vi "TestIntegration.vi"() -> ()   [LabVIEW 2019]
uses:
  ParseVectorFile/Typedefs/PublicEvents--ParseVectorFile.ParsedData.ctl
  Image/SVGImage.lvclass
  ParsePaths/Path.lvclass
  Rectangle/Rectangle.lvclass
  Dot/Dot.lvclass
  PathCommands/Point.ctl
  ParseVectorFile/ParseVectorFile.lvclass
  C:/Program Files (x86)/National Instruments/LabVIEW 2019/vi.lib/JKI/JKI SMO/SMO/SMO.lvclass
  ParsePaths/Path.lvclass/Path.ctl
  ParsePaths/Read Path Commands.vi
  PathCommands/PathCommands.lvclass
  <vilib>/JKI/JKI SMO/SMO/SMO.lvclass
panel:
  out "Points":T1[](array[typedef])
  out "xml string":string
  out "ParsedData":T2
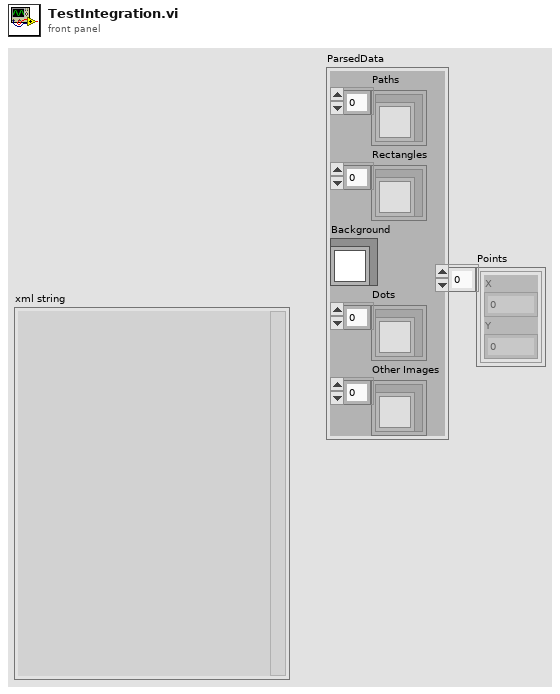
[diagram p1: front panel]
types:
  T1 = typedef "PathCommands.lvclass/Point.ctl" = cluster{"X":dbl, "Y":dbl}
  T2 = typedef "ParseVectorFile.lvclass/PublicEvents--ParseVectorFile.ParsedData.ctl" = cluster{"Paths":refnum<class "Path.lvclass">[], "Rectangles":refnum<class "Rectangle.lvclass">[], "Background":refnum<class "SVGImage.lvclass">, "Dots":refnum<class "Dot.lvclass">[], "Other Images":refnum<class "SVGImage.lvclass">[]}
  T3 = enum16{"open", "replace", "create", "open or create", "replace or create", "replace or create with confirmation"}
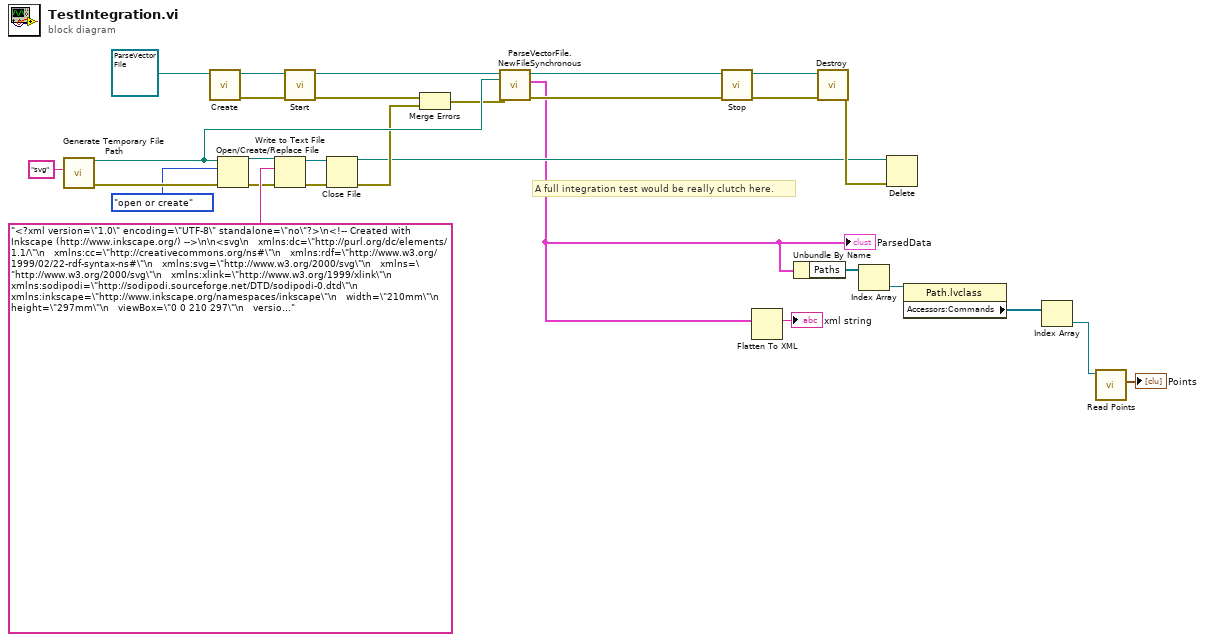
[diagram p0: block diagram]
diagram:
  # "A full integration test would be really clutch here."
  n1 = call <vilib>:"Generate Temporary File Path.vi"("Temporary File Extension (tmp)"="svg") -> ("error out"=w26:errorcluster, "Unique Temporary File Path"=w18:path)  [unwired: 9 in]
  n2 = call <vilib>:"Create.vi"("SMO"=refnum<class "ParseVectorFile.lvclass"> refnum ("ParseVectorFile.lvclass")) -> ("error out"=w14:errorcluster, "SMO out"=w21:refnum<class "ParseVectorFile.lvclass">)  [unwired: 8 in, 1 out]
  n3 = Open/Create/Replace File(file path (use dialog)=w18, error in=w26, operation (0:open)=T3."open or create") -> (refnum out=w24:refnum<file>, error out=w25:errorcluster)  [unwired: 3 in, 1 out]
  n4 = Write to Text File(file (use dialog)=w24, text="<?xml version=\"1.0\" encoding=\"UTF-8\" standalone=\"no\"?>\n<!-- Created with Inkscape (http://www.inkscape.org/) -->\n\n<svg\n   xmlns:dc=\"http://purl.org/dc/elements/1.1/\"\n   xmlns:cc=\"http://creativecommons.org/ns#\"\n   xmlns:rdf=\"http://www.w3.org/1999/02/22-rdf-syntax-ns#\"\n   xmlns:svg=\"http://www.w3.org/2000/svg\"\n   xmlns=\"http://www.w3.org/2000/svg\"\n   xmlns:xlink=\"http://www.w3.org/1999/xlink\"\n   xmlns:sodipodi=\"http://sodipodi.sourceforge.net/DTD/sodipodi-0.dtd\"\n   xmlns:inkscape=\"http://www.inkscape.org/namespaces/inkscape\"\n   width=\"210mm\"\n   height=\"297mm\"\n   viewBox=\"0 0 210 297\"\n   version=\"1.1\"\n   id=\"svg8\"\n   inkscape:version=\"0.92.4 (5da689c313, 2019-01-14)\"\n   sodipodi:docname=\"Rotated Rectangle.svg\">\n  <defs\n     id=\"defs2\" />\n  <sodipodi:namedview\n     id=\"base\"\n     pagecolor=\"#ffffff\"\n     bordercolor=\"#666666\"\n     borderopacity=\"1.0\"\n     inkscape:pageopacity=\"0.0\"\n     inkscape:pageshadow=\"2\"\n     inkscape:zoom=\"1.979899\"\n     inkscape:cx=\"401.06977\"\n     inkscape:cy=\"632.73714\"\n     inkscape:document-units=\"mm\"\n     inkscape:current-layer=\"layer1\"\n     showgrid=\"false\"\n     inkscape:window-width=\"1920\"\n     inkscape:window-height=\"1001\"\n     inkscape:window-x=\"-9\"\n     inkscape:window-y=\"-9\"\n     inkscape:window-maximized=\"1\" />\n  <metadata\n     id=\"metadata5\">\n    <rdf:RDF>\n      <cc:Work\n         rdf:about=\"\">\n        <dc:format>image/svg+xml</dc:format>\n        <dc:type\n           rdf:resource=\"http://purl.org/dc/dcmitype/StillImage\" />\n        <dc:title />\n      </cc:Work>\n    </rdf:RDF>\n  </metadata>\n  <g\n     inkscape:label=\"Layer 1\"\n     inkscape:groupmode=\"layer\"\n     id=\"layer1\">\n    <rect\n       style=\"opacity:1;fill:#00ff00;fill-opacity:1;stroke:#000000;stroke-width:0.2;stroke-miterlimit:4;stroke-dasharray:none;stroke-opacity:1\"\n       id=\"rect10\"\n       width=\"10.1\"\n       height=\"10.2\"\n       x=\"-10.3\"\n       y=\"10.4\"\n       transform=\"rotate(-10.5)\" />\n    <rect\n       style=\"opacity:1;fill:#00ff00;fill-opacity:1;stroke:#000000;stroke-width:0.2;stroke-miterlimit:4;stroke-dasharray:none;stroke-opacity:1\"\n       id=\"rect12\"\n       width=\"10.6\"\n       height=\"10.7\"\n       x=\"-10.8\"\n       y=\"10.9\"\n       inkscape:transform-center-x=\"33.251622\"\n       inkscape:transform-center-y=\"66.085109\"\n       transform=\"rotate(-11.1)\" />\n    <image\n       sodipodi:absref=\"C:\\gold_75nm_low_voltage.png\"\n       y=\"100.1\"\n       x=\"100\"\n       id=\"image33\"\n       xlink:href=\"file:///C:/gold_75nm_low_voltage.png\"\n       preserveAspectRatio=\"none\"\n       height=\"70.1\"\n       width=\"70\" />\n    <path\n       style=\"fill:none;stroke:#45fc03;stroke-width:0.123456789px;stroke-linecap:butt;stroke-linejoin:miter;stroke-opacity:1\"\n       d=\"m 1.1,1.2 c 1.3,1.4 1.5,-1.6 1.7,-1.8 1.9,1.10 1.11,1.12 1.13,1.14 0,0 1.15,1.16 1.17,1.18 -1.19,1.20 -1.21,-1.22 -1.23,-1.24 0,0 -1.25,-1.26 -1.27,-1.28\"\n       id=\"path58\"\n       inkscape:connector-curvature=\"0\" />\n    <path\n       style=\"fill:none;stroke:#000000;stroke-width:0.1234px;stroke-linecap:butt;stroke-linejoin:miter;stroke-opacity:1\"\n       d=\"m 159.42627,92.271539 41.29314,-4.677214 c 0,0 -1.87088,4.409945 -4.54358,22.717905 -2.6727,18.30797 -40.09043,-17.773419 -40.09043,-17.773419 l -32.60688,-0.668174\"\n       id=\"path60\"\n       inkscape:connector-curvature=\"0\" />\n  </g>\n</svg>", error in=w25) -> (refnum out=w20:refnum<file>, error out=w28:errorcluster)  [unwired: 1 in, 1 out]
  n5 = call <vilib>:"Start.vi"("error in (no error)"=w14, "SMO"=w21) -> ("error out"=w15:errorcluster, "SMO out"=w19:refnum<class "ParseVectorFile.lvclass">)  [unwired: 8 in]
  n6 = Close File(refnum=w20, error in=w28) -> (path=w8:path, error out=w13:errorcluster)
  n7 = Merge Errors(w15, w13) -> (w12:errorcluster)
  n8 = call "ParseVectorFile.NewFileSynchronous.vi"("error in (no error)"=w12, "Path"=w18, "ParseVectorFile"=w19) -> ("error out"=w11:errorcluster, "ParsedData"=w6:T2, "ParseVectorFile out"=w17:refnum<class "ParseVectorFile.lvclass">)  [unwired: 6 in]
  "ParsedData" <- w6
  n9 = call <vilib>:"Stop.vi"("error in (no error)"=w11, "SMO"=w17) -> ("error out"=w10:errorcluster, "SMO out"=w16:refnum<class "ParseVectorFile.lvclass">)  [unwired: 8 in]
  n10 = Flatten To XML(anything=w6) -> (xml string=→"xml string":string)
  n11 = Unbundle By Name(w6) -> ("Paths"=w5:refnum<class "Path.lvclass">[])
  n12 = call <vilib>:"Destroy.vi"("error in (no error)"=w10, "SMO"=w16) -> ("error out"=w9:errorcluster)  [unwired: 9 in]
  n13 = Index Array(array=w5) -> (element=w4:refnum<class "Path.lvclass">)  [unwired: 1 in]
  n14 = Delete(path (use dialog)=w8, error in=w9) -> ()  [unwired: 3 in, 3 out]
  n15 = property class="Path.lvclass"(reference=w4) -> ("Accessors:Commands"=w3:refnum<class "PathCommands.lvclass">[])  [unwired: 1 in, 2 out]
  n16 = Index Array(array=w3) -> (element=w2:refnum<class "PathCommands.lvclass">)  [unwired: 1 in]
  n17 = call-dynamic "Read Points.vi"("PathCommands in"=w2) -> ("Points"=→"Points":T1[])  [unwired: 8 in, 2 out]
